vi "Connection Offsets Display.vi"() -> ()   [LabVIEW 2009]
uses:
  lib/Launcher/Launcher Actions.ctl
  lib/Launcher/NoPanelAppTypes.ctl
  lib/Data Access Objects/Metadata/Persistant DAO Actions.ctl
  lib/Data Access Objects/Metadata/DAO Actions.ctl
panel:
  in  "Tab Control":enum32{"Readings", "Offsets"}(tab)
  out "LBCB 1 Data":dbl[][](array[numeric])
  out "LBCB 2 Data":dbl[][](array[numeric])
  out "L1 Connection Offset":dbl[][](array[numeric])
  out "L2 Connection Offset":dbl[][](array[numeric])
  out "DOF Labels 2":string[](array[string])=["Dx", "Dy", "Dz", "Rx", "Ry", "Rz"]
  out "DOF Labels":string[](array[string])=["Dx", "Dy", "Dz", "Rx", "Ry", "Rz"]
  in  "Ok":bool
  # "LBCB 1"
  # "LBCB 2"
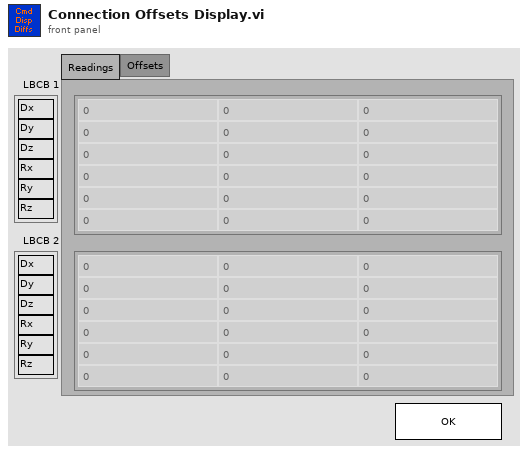
[diagram p1: front panel]
types:
  T1 = typedef "NoPanelAppTypes.ctl" = enum16{"NTCP Socket", "Data Archiving", "DAQ Link", "Control Loops", "Cmd Disp Diffs", "Connection Offsets", "Limits", "Increment Limits"}
  T2 = typedef "Launcher Actions.ctl" = enum16{"Launch", "Stop All", "Stop", "Kill", "Running?", "Init"}
  T3 = typedef "DAO Actions.ctl" = enum16{"Init", "Get", "Set"}
  T4 = typedef "Persistant DAO Actions.ctl" = enum16{"Init", "Get", "Set", "Load", "Save"}
  T5 = typedef "Cartesian Point.ctl" = cluster{"Dx":dbl, "Dy":dbl, "Dz":dbl, "Rx":dbl, "Ry":dbl, "Rz":dbl}
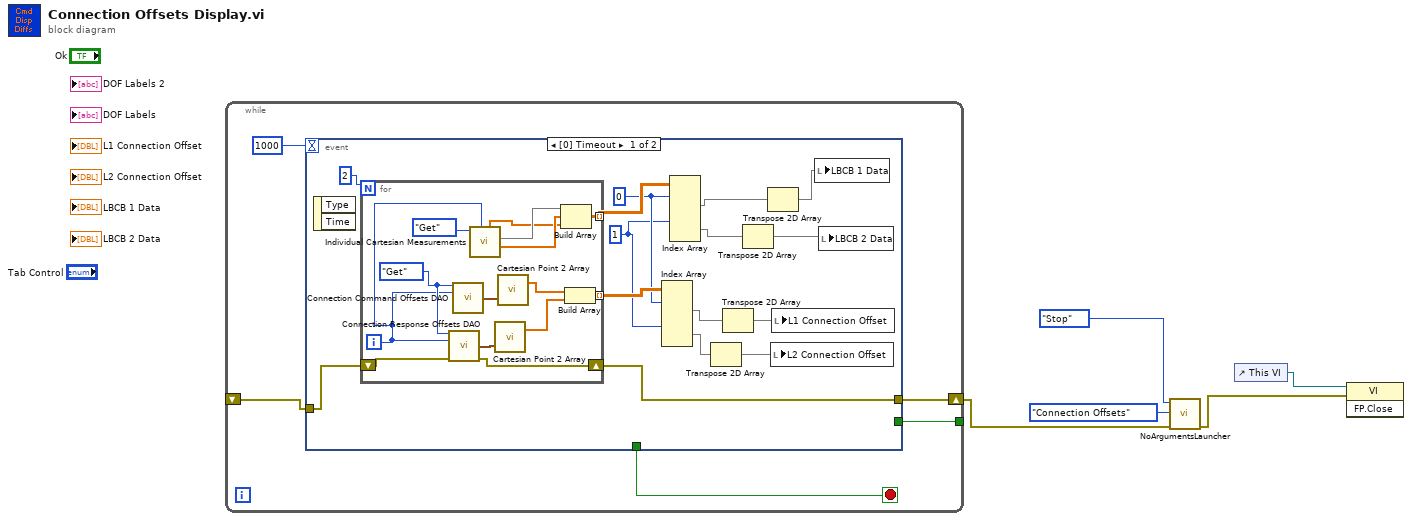
[diagram p0: block diagram]
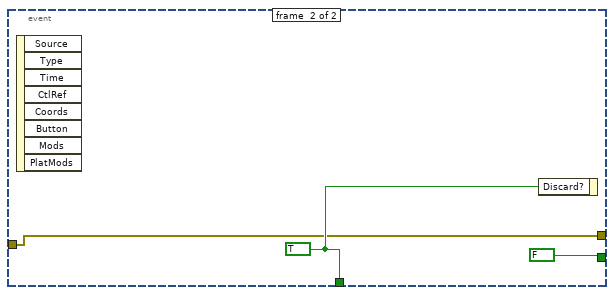
[diagram p2: hidden frame]
diagram:
  n1 = while {
    tunnel: [w8] -> _
    shift-right: [w6] -> w5
    shift-left: _ -> [w7]
    stop <- w9 stop-if-true
    n2 = event shown="[0] Timeout" {
      selector: _ -> [_ _]
      dyn-events: _ -> [_ _]
      timeout: 1000 -> [_ _]
      tunnel: [_ w41] -> w9
      tunnel: [_ FALSE] -> w8
      tunnel: w7 -> [w25 w40]
      tunnel: [w24 w40] -> w6
      event #0 {
        w15 = 1 ("index (page)")
        w16 = 0 ("index (page)")
        n3 = event-data() -> ()  [unwired: 3 out]
        n4 = for {
          N: 2 -> [_]
          shift-right: [w36] -> w24
          shift-left: w25 -> [w37]
          tunnel: [w27] -> w22 mode=indexing
          tunnel: [w26] -> w19 mode=indexing
          i -> [w33]
          w39 = Persistant_DAO_Actions."Get" ("Actions")
          n5 = call "Connection Response Offsets DAO.vi"("Actions"=w39, "LBCB Number"=w33, "error in (no error)"=w37) -> ("Offsets Out"=w34:T5, "error out"=w36:errorcluster)  [unwired: 10 in, 1 out]
          n6 = call "Connection Command Offsets DAO.vi"("Actions"=w39, "LBCB Number"=w33) -> ("Offsets Out"=w35:T5)  [unwired: 11 in, 2 out]
          n7 = call "Individual Cartesian Measurements.vi"("LBCB Number"=w33, "DAO Actions"=DAO_Actions."Get") -> ("Displacements Out"=w31:dbl[], 2:w32, "Forces Out"=w30:dbl[])  [unwired: 6 in, 1 out]
          n8 = call "Cartesian Point 2 Array.vi"("Cart Disp"=w34) -> ("Array"=w28:dbl[])  [unwired: 2 in]
          n9 = call "Cartesian Point 2 Array.vi"("Cart Disp"=w35) -> ("Array"=w29:dbl[])  [unwired: 2 in]
          n10 = Build Array(w32, w31, w30) -> (w27:dbl[][])
          n11 = Build Array(w29, w28) -> (w26:dbl[][])
        }
        n12 = Index Array(array=w19, index (dim 0) #1=w16, index (dim 0) #2=w15) -> (element #1=w18:dbl[][], element #2=w17:dbl[][])  [unwired: 4 in]
        n13 = Index Array(array=w22, index (dim 0) #1=w16, index (dim 0) #2=w15) -> (element #1=w21:dbl[][], element #2=w20:dbl[][])  [unwired: 4 in]
        n14 = Transpose 2D Array(2D array=w17) -> (transposed array=w11:dbl[][])
        n15 = Transpose 2D Array(2D array=w18) -> (transposed array=w12:dbl[][])
        n16 = Transpose 2D Array(2D array=w20) -> (transposed array=w13:dbl[][])
        n17 = Transpose 2D Array(2D array=w21) -> (transposed array=w14:dbl[][])
        n18 = local write "L2 Connection Offset"(w11) -> ()
        n19 = local write "L1 Connection Offset"(w12) -> ()
        n20 = local write "LBCB 1 Data"(w14) -> ()
        n21 = local write "LBCB 2 Data"(w13) -> ()
      }
      event #1 {
        w41 = TRUE
        n22 = event-data() -> ()  [unwired: 9 out]
        n23 = event-data("Discard?"=w41) -> ()  [unwired: 1 in, 1 out]
      }
    }
  }
  n24 = call "NoArgumentsLauncher.vi"("error in (no error)"=w5, "Application"=NoPanelAppTypes."Connection Offsets", "Application Launcher Actions"=Launcher_Actions."Stop") -> ("error out"=w1:errorcluster)  [unwired: 8 out]
  n25 = control-ref of="This VI"() -> (w4:refnum<vi>)
  n26 = invoke class="VI" method="FP.Close"(reference=w4, error in=w1) -> ()  [unwired: 1 in, 3 out]
